vi "VI Tree.vi"   [LabVIEW 2010, in "Eurotherm 32xx Series.lvlib"]
doc: "This is the instrument driver for the <B>Eurotherm 32xx Series</B>. The VI Tree displays all the user-callable VIs of the instrument driver in an organized table."
uses:
  <instrlib>/Eurotherm 32xx Series/Eurotherm 32xx Series.lvlib
panel:
  # "(c) 2010 <Invensys Eurotherm>.  ALL RIGHTS RESERVED."
  # "SEE DIAGRAM\nFOR VI TREE."
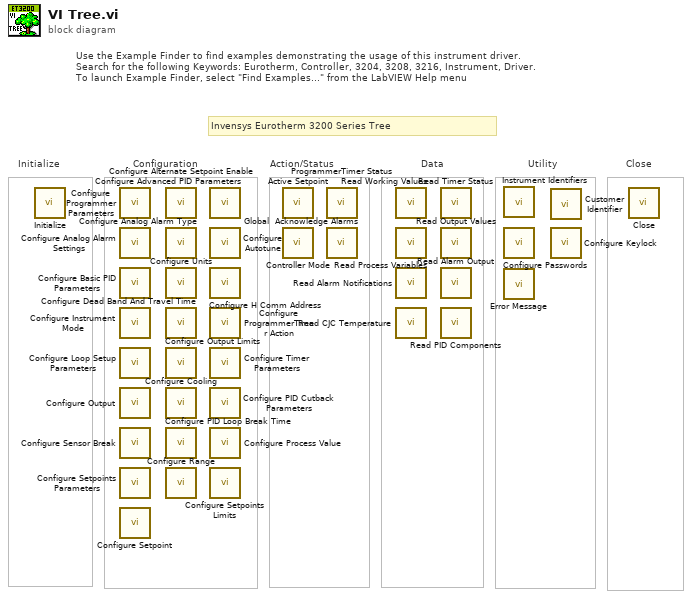
[diagram p0: block diagram]
diagram:
  # "Invensys Eurotherm 3200 Series Tree"
  # "Use the Example Finder to find examples demonstrating the usage of this instrument driver.\nSearch for the following Keywords: Eurotherm, Controller, 3204, 3208, 3216, Instrument, Driver.\nTo launch Example Finder, select \"Find Examples...\" from the LabVIEW Help menu"
  # "Configuration"
  # "Utility"
  # "Data"
  # "Action/Status"
  # "Close"
  # "Initialize"
  n1 = call <instrlib>:"Initialize.vi"() -> ()  [unwired: 14 in, 2 out]
  n2 = call <instrlib>:"Configure Programmer Parameters.vi"() -> ()  [unwired: 14 in, 2 out]
  n3 = call <instrlib>:"Configure Analog Alarm Settings.vi"() -> ()  [unwired: 14 in, 2 out]
  n4 = call <instrlib>:"Configure Basic PID Parameters.vi"() -> ()  [unwired: 14 in, 2 out]
  n5 = call <instrlib>:"Configure Instrument Mode.vi"() -> ()  [unwired: 14 in, 2 out]
  n6 = call <instrlib>:"Configure Loop Setup Parameters.vi"() -> ()  [unwired: 14 in, 2 out]
  n7 = call <instrlib>:"Configure Output.vi"() -> ()  [unwired: 14 in, 2 out]
  n8 = call <instrlib>:"Configure Sensor Break.vi"() -> ()  [unwired: 14 in, 2 out]
  n9 = call <instrlib>:"Configure Setpoints Parameters.vi"() -> ()  [unwired: 14 in, 2 out]
  n10 = call <instrlib>:"Configure Setpoint.vi"() -> ()  [unwired: 14 in, 2 out]
  n11 = call <instrlib>:"Configure Alternate Setpoint Enable.vi"() -> ()  [unwired: 14 in, 2 out]
  n12 = call <instrlib>:"Configure Analog Alarm Type.vi"() -> ()  [unwired: 14 in, 2 out]
  n13 = call <instrlib>:"Configure Units.vi"() -> ()  [unwired: 14 in, 2 out]
  n14 = call <instrlib>:"Configure Dead Band And Travel Time.vi"() -> ()  [unwired: 14 in, 2 out]
  n15 = call <instrlib>:"Configure Output Limits.vi"() -> ()  [unwired: 14 in, 2 out]
  n16 = call <instrlib>:"Configure Cooling.vi"() -> ()  [unwired: 14 in, 2 out]
  n17 = call <instrlib>:"Configure PID Loop Break Time.vi"() -> ()  [unwired: 14 in, 2 out]
  n18 = call <instrlib>:"Configure Range.vi"() -> ()  [unwired: 14 in, 2 out]
  n19 = call <instrlib>:"Configure Advanced PID Parameters.vi"() -> ()  [unwired: 14 in, 2 out]
  n20 = call <instrlib>:"Configure Autotune.vi"() -> ()  [unwired: 14 in, 2 out]
  n21 = call <instrlib>:"Configure H Comm Address.vi"() -> ()  [unwired: 14 in, 2 out]
  n22 = call <instrlib>:"Configure ProgrammerTimer Action.vi"() -> ()  [unwired: 14 in, 2 out]
  n23 = call <instrlib>:"Configure Timer Parameters.vi"() -> ()  [unwired: 14 in, 2 out]
  n24 = call <instrlib>:"Configure PID Cutback Parameters.vi"() -> ()  [unwired: 14 in, 2 out]
  n25 = call <instrlib>:"Configure Process Value.vi"() -> ()  [unwired: 14 in, 2 out]
  n26 = call <instrlib>:"Configure Setpoints Limits.vi"() -> ()  [unwired: 14 in, 2 out]
  n27 = call <instrlib>:"Active Setpoint.vi"() -> ()  [unwired: 14 in, 2 out]
  n28 = call <instrlib>:"Controller Mode.vi"() -> ()  [unwired: 14 in, 2 out]
  n29 = call <instrlib>:"ProgrammerTimer Status.vi"() -> ()  [unwired: 14 in, 2 out]
  n30 = call <instrlib>:"Global  Acknowledge Alarms.vi"() -> ()  [unwired: 14 in, 2 out]
  n31 = call <instrlib>:"Read Working Values.vi"() -> ()  [unwired: 12 in, 4 out]
  n32 = call <instrlib>:"Read Process Variables.vi"() -> ()  [unwired: 12 in, 4 out]
  n33 = call <instrlib>:"Read Alarm Notifications.vi"() -> ()  [unwired: 13 in, 3 out]
  n34 = call <instrlib>:"Read CJC Temperature.vi"() -> ()  [unwired: 13 in, 3 out]
  n35 = call <instrlib>:"Read Timer Status.vi"() -> ()  [unwired: 13 in, 3 out]
  n36 = call <instrlib>:"Read Output Values.vi"() -> ()  [unwired: 13 in, 3 out]
  n37 = call <instrlib>:"Read Alarm Output.vi"() -> ()  [unwired: 13 in, 3 out]
  n38 = call <instrlib>:"Read PID Components.vi"() -> ()  [unwired: 11 in, 5 out]
  n39 = call <instrlib>:"Instrument Identifiers.vi"() -> ()  [unwired: 10 in, 6 out]
  n40 = call <instrlib>:"Configure Passwords.vi"() -> ()  [unwired: 14 in, 2 out]
  n41 = call <instrlib>:"Error Message.vi"() -> ()  [unwired: 11 in, 5 out]
  n42 = call <instrlib>:"Customer Identifier.vi"() -> ()  [unwired: 14 in, 2 out]
  n43 = call <instrlib>:"Configure Keylock.vi"() -> ()  [unwired: 14 in, 2 out]
  n44 = call <instrlib>:"Close.vi"() -> ()  [unwired: 15 in, 1 out]
